vi "error_comparison.vi"(9 "epsilon":i32 min=0 max=10, 10 "measurement":i32 min=0 max=10, 11 "setpoint":i32 min=0 max=10) -> (3 "output":i32 min=0 max=10)   [LabVIEW 2014]
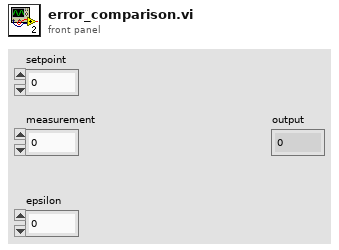
[diagram p1: front panel]
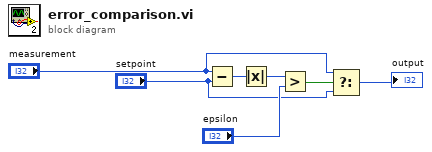
[diagram p0: block diagram]
diagram:
  n1 = Subtract(x="measurement", y="setpoint") -> (x-y=w7:i32)
  n2 = Absolute Value(x=w7) -> (abs(x)=w6:i32)
  n3 = Greater?(x=w6, y="epsilon") -> (0:w5:bool)
  n4 = Select(t="measurement", s=w5, f="setpoint") -> (s? t:f=→"output":i32)
